vi "SPI Master and Slave with debug and disconnect [FPGA].vi"() -> ()   [LabVIEW 2011]
uses:
  <vilib>/Platform/TimedLoop/XDataNode/timing_clust.ctl
  <vilib>/Platform/TimedLoop/XDataNode/nitl_modes.ctl
  <vilib>/Platform/TimedLoop/XDataNode/wakeup.ctl
  SPI Slave State.ctl
  SPI Master State.ctl
  <vilib>/rvi/interface/RandomDataEmulation/nirviRandomDataFPGAFIFO.vi
  <vilib>/rvi/interface/RandomDataEmulation/niFpgaRandomDataHandleErrors.vi
  <vilib>/Platform/TimedLoop/XDataNode/XDataNode.xnode
  <vilib>/rvi/DataTransferAndStorage/Container/XNode/niFpgaContainer.xnode
  <vilib>/rvi/interface/RandomDataEmulation/nirviRandomDataFpgaReadWriteTemplate.vi
  <vilib>/Platform/TimedLoop/XDataNode/XDNodeRunTimeDep.lvlib
panel:
  in  "Disconnect Master and Slave":bool
  out "Slave Data Out":u32
  in  "Slave Data In":u32
  in  "Data Length":u8
  in  "HCP-1":u8
  out "Data Out":u32
  in  "Data In":u32
  in  "TX":bool
  in  "CPOL":bool
  in  "CPHA":bool
  in  "RESET":bool
  out "_SS":bool
  out "SCLK":bool
  out "MOSI":bool
  out "MISO":bool
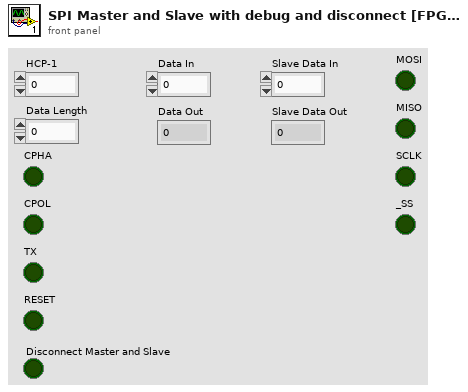
[diagram p1: front panel]
types:
  T1 = typedef "XDNodeRunTimeDep.lvlib/timing_clust.ctl" = cluster{"Expected End [f-1]":u64, "Actual End [f-1]":u64, "Finished Late? [f-1]":bool, "Expected End [i-1]":u64, "Actual End [i-1]":u64, "Finished Late? [i-1]":bool, "Expected Start [i]":u64, "Actual Start [i]":u64, "Expected Start [f]":u64, "Actual Start [f]":u64, "Source Name":string, "Structure Name":string, "Period":i64, "Deadline":i64, "Offset":i64, "Start":i64, "Priority":i32, "Timeout":i32, "Mode":T2, "Wakeup Reason":T3, "Error":errorcluster, "Source Type":string, "Secondary Source Type":string, "Global End Time":u64, "Global Start Time":u64, "Frame Duration":u64, "Iteration Duration":u64, "Assigned CPU":i32, "I/O Scan Engine Mode":u32}
  T2 = typedef "XDNodeRunTimeDep.lvlib/nitl_modes.ctl" = enum32{"No Change", "Process missed periods, maintain original phase", "Discard missed periods, maintain original phase", "Process missed periods, ignore original phase", "Discard missed periods, ignore original phase"}
  T3 = typedef "XDNodeRunTimeDep.lvlib/wakeup.ctl" = enum32{"Normal", "Aborted", "Asynchronous wakeup", "Timing source error", "Timed loop error", "Timeout"}
  T4 = typedef "SPI Slave State.ctl" = enum8{"RESET", "Wait for _SS", "Assert MISO", "Latch MOSI"}
  T5 = typedef "SPI Master State.ctl" = enum8{"RESET", "Wait for TX", "Assert MOSI", "Toggle SCLK", "Latch MISO and Toggle SCLK", "Assert MOSI and Toggle SCLK"}
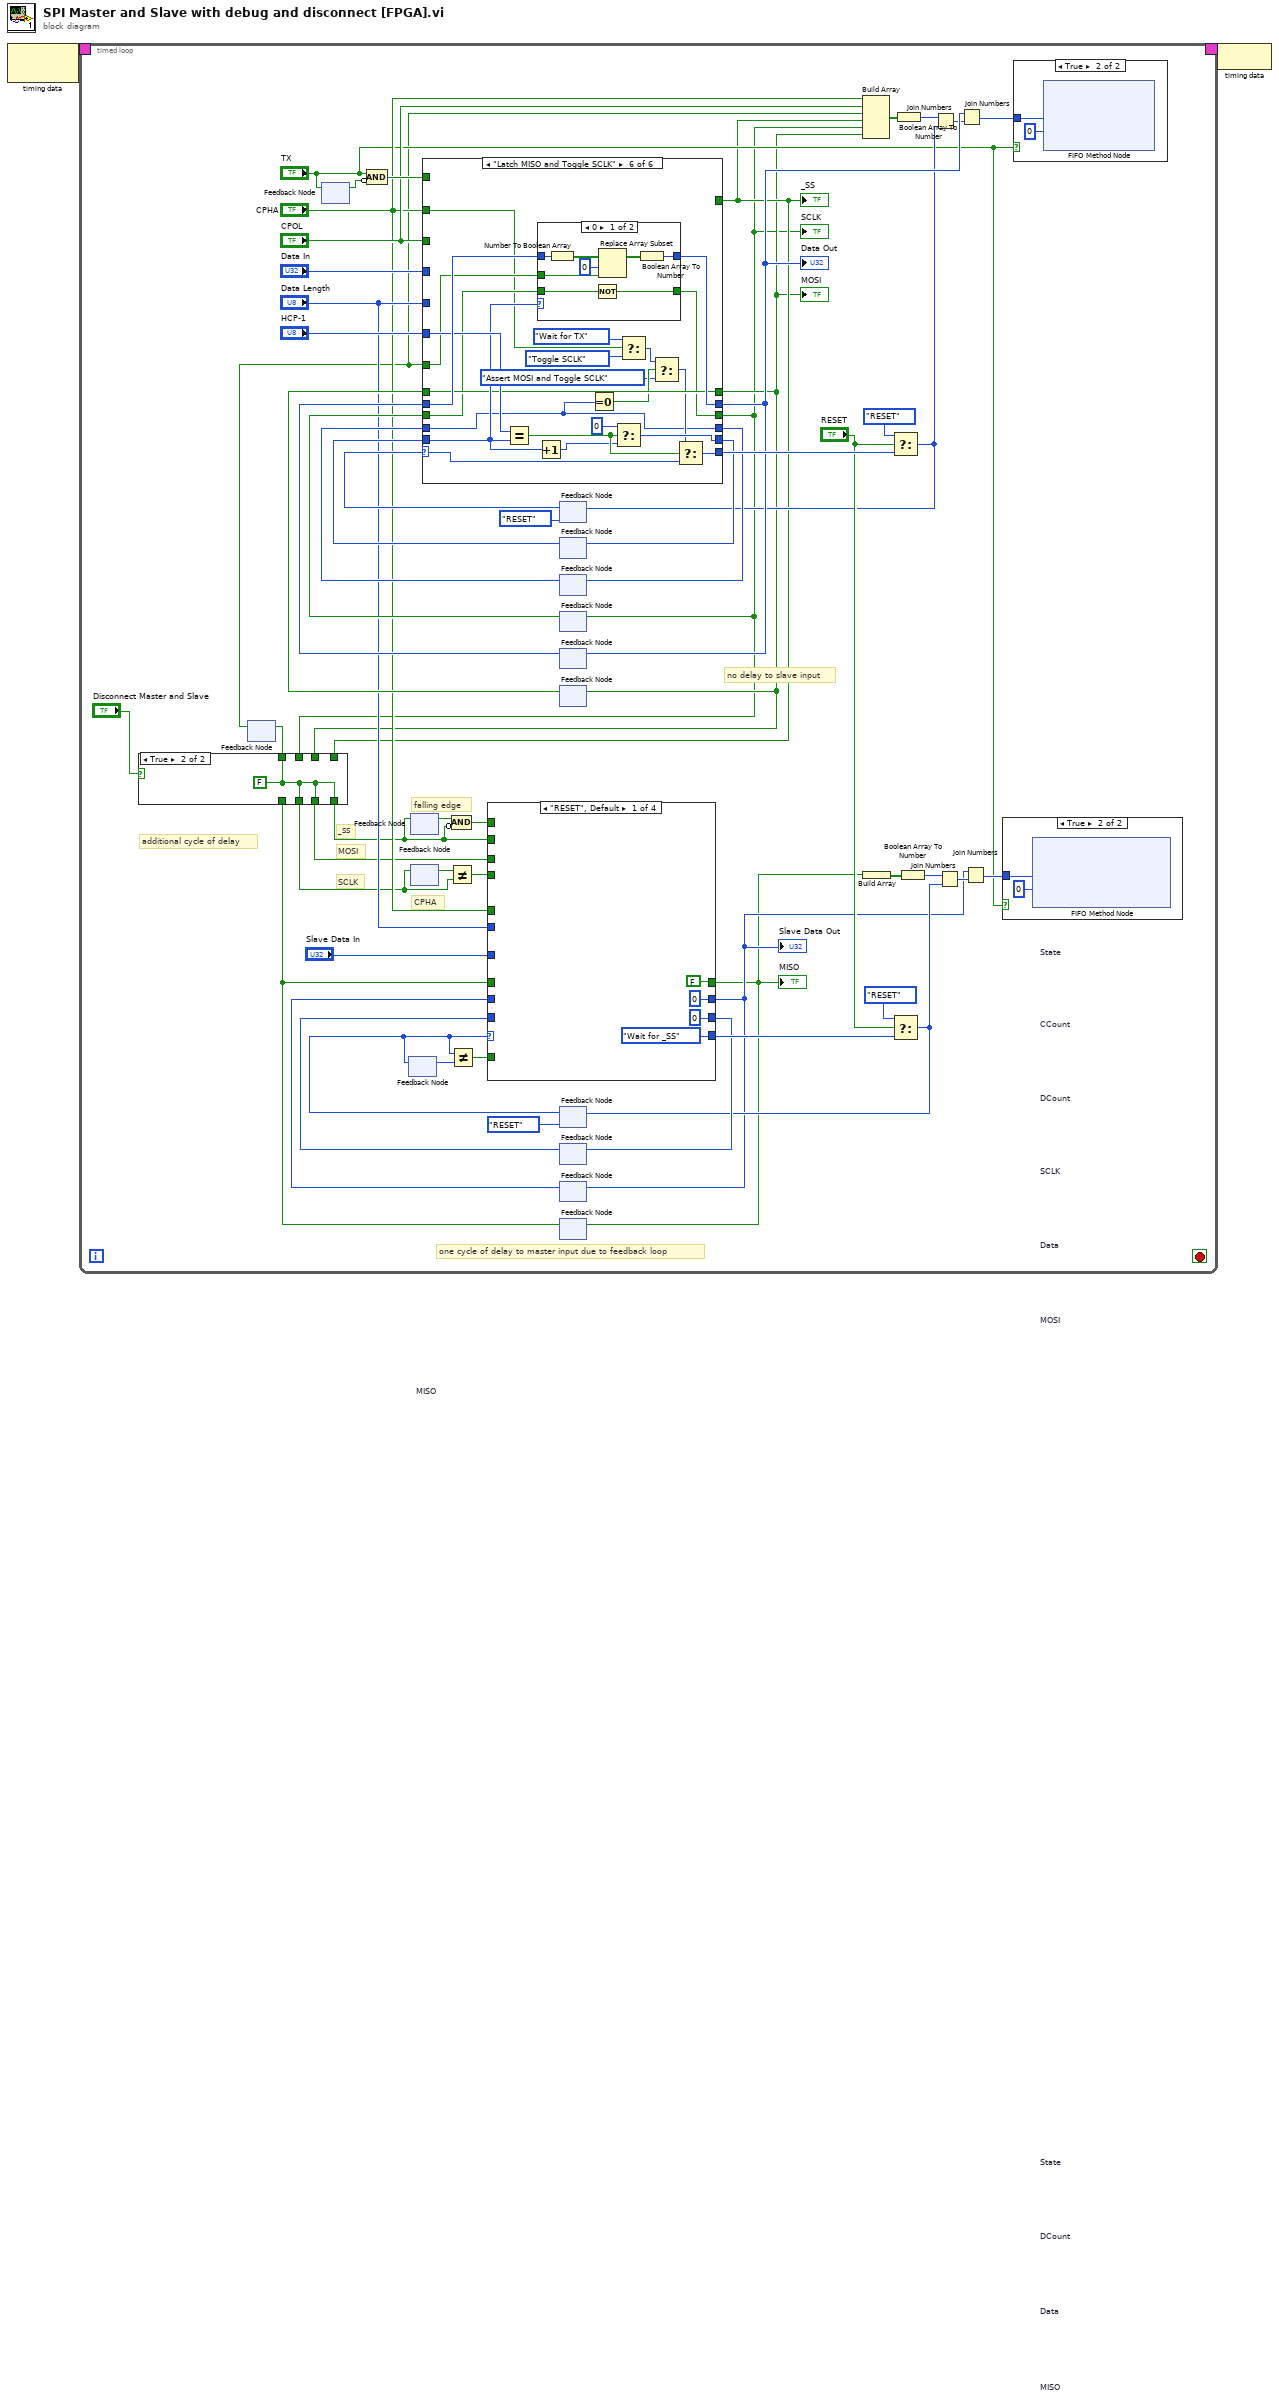
[diagram p0: block diagram]
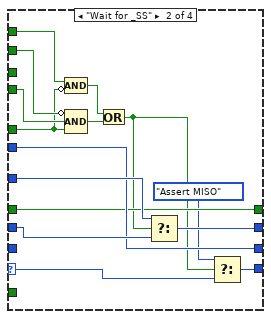
[diagram p4: hidden frame]
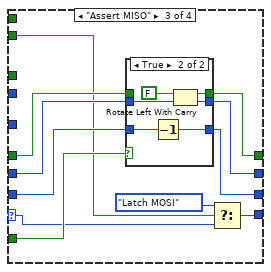
[diagram p5: hidden frame]
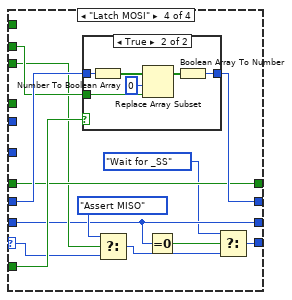
[diagram p7: hidden frame]
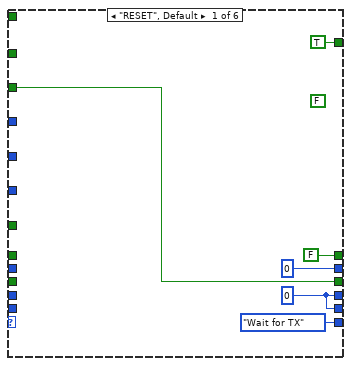
[diagram p10: hidden frame]
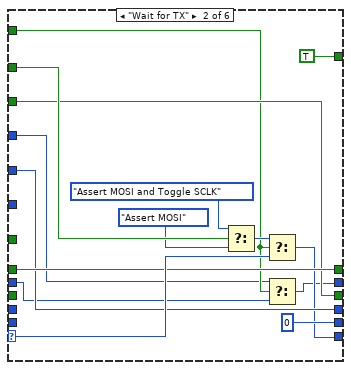
[diagram p11: hidden frame]
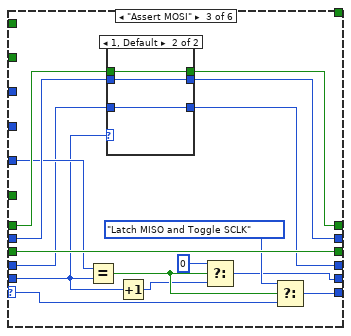
[diagram p12: hidden frame]
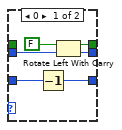
[diagram p13: hidden frame]
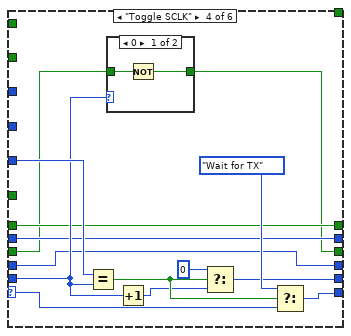
[diagram p14: hidden frame]
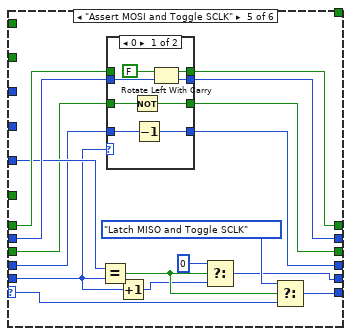
[diagram p16: hidden frame]
diagram:
  n1 = node-c288() -> (w2:T1)  [unwired: 1 in]
  n2 = timed-loop {
    timing: w2 -> [_]
    timing-out: [_] -> w1
    stop <- _ stop-if-true
    # "additional cycle of delay"
    # "CPHA"
    # "falling edge"
    # "SCLK"
    # "MOSI"
    # "_SS"
    # "one cycle of delay to master input due to feedback loop"
    # "no delay to slave input"
    n3 = feedback #1 "MISO"() -> (w7:bool)  [unwired: 1 in]
    n4 = feedback #2() -> (w55:bool)  [unwired: 1 in]
    n5 = feedback-in #2("TX") -> ()
    n6 = Compound Arithmetic op=AND("TX", invert w55) -> (w47:bool)
    n7 = feedback #3 ("State")() -> (w23:T4)  [unwired: 1 in]
    n8 = feedback #4() -> (w27:bool)  [unwired: 1 in]
    n9 = feedback #5() -> (w25:bool)  [unwired: 1 in]
    n10 = feedback #6 "State"(SPI_Master_State."RESET") -> (w58:T5)
    n11 = feedback #7 "CCount"() -> (w52:u8)  [unwired: 1 in]
    n12 = feedback #8 "DCount"() -> (w51:u8)  [unwired: 1 in]
    n13 = feedback #9 "SCLK"() -> (w50:bool)  [unwired: 1 in]
    n14 = feedback #10 "Data"() -> (w48:u32)  [unwired: 1 in]
    n15 = feedback #11 "MOSI"() -> (w46:bool)  [unwired: 1 in]
    n16 = case shown="\"Latch MISO and Toggle SCLK\"" w58 {
      selector: w58 -> [_ w145 w157 w185 w201 w237]
      tunnel: [SPI_Master_State."Wait for TX" w138 w158 w186 w202 w238] -> w57
      tunnel: w47 -> [_ w137 _ _ _ _]
      tunnel: [w132 u8 0 w151 w179 w195 w232] -> w54
      tunnel: [w132 w140 w149 w178 w191 w220] -> w53
      tunnel: w52 -> [_ _ w154 w182 w198 w235]
      tunnel: w51 -> [_ _ w150 w178 w192 w220]
      tunnel: [TRUE ("MOSI") TRUE ("MOSI") _ _ _ _] -> w12
      tunnel: "CPHA" -> [_ w146 _ _ _ w226]
      tunnel: [w130 w139 w160 w174 w193 w228] -> w10
      tunnel: "CPOL" -> [w130 w139 _ _ _ _]
      tunnel: w50 -> [_ _ w160 w175 w194 w229]
      tunnel: "Data In" -> [_ w136 _ _ _ _]
      tunnel: [u32 0 ("Data In") w134 w163 w177 w206 w240] -> w40
      tunnel: w48 -> [_ w135 w164 w177 w207 w241]
      tunnel: "HCP-1" -> [_ _ w159 w187 w203 w239]
      tunnel: w7 -> [_ _ _ _ _ w230]
      tunnel: "Data Length" -> [_ w140 _ _ _ _]
      tunnel: [FALSE ("msb carry out") w141 w162 w176 w205 w231] -> w11
      tunnel: w46 -> [_ w141 w161 w176 w204 w231]
      frame "RESET", Default {
        (unwired) FALSE ("msb carry out")
        w132 = u8 0
      }
      frame "Wait for TX" {
        n17 = Select(t=SPI_Master_State."Assert MOSI and Toggle SCLK", s=w146, f=SPI_Master_State."Assert MOSI" ("t")) -> (s? t:f=w142:T5)
        n18 = Select(t=w142, s=w137, f=w145) -> (s? t:f=w138:T5)
        n19 = Select(t=w136, s=w137, f=w135) -> (s? t:f=w134:u32)
      }
      frame "Assert MOSI" {
        n20 = Equal?(x=w159, y=w154) -> (x = y?=w155:bool)
        n21 = case shown="1, Default" w154 {
          tunnel: w164 -> [w169 w172]
          tunnel: [w168 w172] -> w163
          tunnel: [w167 w173] -> w162
          tunnel: w161 -> [_ w173]
          tunnel: w150 -> [w166 w171]
          tunnel: [w165 w171] -> w149
          frame 0 {
            n22 = Decrement(x=w166) -> (x-1=w165:u8)
            n23 = Rotate Left With Carry(2:w169, 3:FALSE ("carry")) -> (0:w168:u32, 1:w167:bool)
          }
          frame 1, Default {
          }
        }
        n24 = Increment(x=w154) -> (x+1=w153:u8)
        n25 = Select(t=u8 0, s=w155, f=w153) -> (s? t:f=w151:u8)
        n26 = Select(t=SPI_Master_State."Latch MISO and Toggle SCLK", s=w155, f=w157) -> (s? t:f=w158:T5)
      }
      frame "Toggle SCLK" {
        n27 = Equal?(x=w187, y=w182) -> (x = y?=w183:bool)
        n28 = case shown="0" w182 {
          tunnel: w175 -> [w189 w190]
          tunnel: [w188 w190] -> w174
          frame 0 {
            n29 = Not(x=w189) -> (.not. x?=w188:bool)
          }
          frame 1, Default {
          }
        }
        n30 = Increment(x=w182) -> (x+1=w181:u8)
        n31 = Select(t=u8 0, s=w183, f=w181) -> (s? t:f=w179:u8)
        n32 = Select(t=SPI_Master_State."Wait for TX", s=w183, f=w185) -> (s? t:f=w186:T5)
      }
      frame "Assert MOSI and Toggle SCLK" {
        n33 = Equal?(x=w203, y=w198) -> (x = y?=w199:bool)
        n34 = case shown="0" w198 {
          tunnel: w207 -> [w214 w218]
          tunnel: [w213 w218] -> w206
          tunnel: [w212 w219] -> w205
          tunnel: w204 -> [_ w219]
          tunnel: w194 -> [w211 w217]
          tunnel: [w210 w217] -> w193
          tunnel: w192 -> [w209 w216]
          tunnel: [w208 w216] -> w191
          frame 0 {
            n35 = Not(x=w211) -> (.not. x?=w210:bool)
            n36 = Decrement(x=w209) -> (x-1=w208:u8)
            n37 = Rotate Left With Carry(2:w214, 3:FALSE ("carry")) -> (0:w213:u32, 1:w212:bool)
          }
          frame 1, Default {
          }
        }
        n38 = Increment(x=w198) -> (x+1=w197:u8)
        n39 = Select(t=u8 0, s=w199, f=w197) -> (s? t:f=w195:u8)
        n40 = Select(t=SPI_Master_State."Latch MISO and Toggle SCLK", s=w199, f=w201) -> (s? t:f=w202:T5)
      }
      frame "Latch MISO and Toggle SCLK" {
        n41 = Equal?(x=w239, y=w235) -> (x = y?=w236:bool)
        n42 = Increment(x=w235) -> (x+1=w234:u8)
        n43 = case shown="0" w235 {
          tunnel: w241 -> [w249 w251]
          tunnel: [w244 w251] -> w240
          tunnel: w230 -> [w247 _]
          tunnel: w229 -> [w243 w250]
          tunnel: [w242 w250] -> w228
          frame 0 {
            n44 = Number To Boolean Array(number=w249) -> (Boolean array=w248:bool[])
            n45 = Not(x=w243) -> (.not. x?=w242:bool)
            n46 = Replace Array Subset(array=w248, new element=w247, index=0) -> (w245:bool[])
            n47 = Boolean Array To Number(Boolean array=w245) -> (number=w244:u32)
          }
          frame 1, Default {
          }
        }
        n48 = Equal To 0?(x=w220) -> (x = 0?=w227:bool)
        n49 = Select(t=u8 0, s=w236, f=w234) -> (s? t:f=w232:u8)
        n50 = Select(t=SPI_Master_State."Wait for TX", s=w226, f=SPI_Master_State."Toggle SCLK" ("t")) -> (s? t:f=w222:T5)
        n51 = Select(t=w222, s=w227, f=SPI_Master_State."Assert MOSI and Toggle SCLK" ("t")) -> (s? t:f=w224:T5)
        n52 = Select(t=w224, s=w236, f=w237) -> (s? t:f=w238:T5)
      }
    }
    "SCLK" <- w10
    "_SS" <- w12
    "MOSI" <- w11
    "Data Out" <- w40
    n53 = feedback-in #7(w54) -> ()
    n54 = feedback-in #8(w53) -> ()
    n55 = feedback-in #9(w10) -> ()
    n56 = feedback-in #10(w40) -> ()
    n57 = feedback-in #11(w11) -> ()
    n58 = feedback #12 "State"(SPI_Slave_State."RESET" ("SPI Slave State")) -> (w22:T4)
    n59 = feedback-in #3(w22) -> ()
    n60 = Not Equal?(x=w22, y=w23) -> (x != y?=w21:bool)
    n61 = feedback #13 "DCount"() -> (w34:u8)  [unwired: 1 in]
    n62 = feedback #14 "Data"() -> (w31:u32)  [unwired: 1 in]
    n63 = feedback #15 "MISO"() -> (w9:bool)  [unwired: 1 in]
    n64 = case shown="True" "Disconnect Master and Slave" {
      tunnel: w12 -> [w63 _]
      tunnel: [w63 w64] -> w4
      tunnel: w11 -> [w62 _]
      tunnel: [w62 w64] -> w5
      tunnel: w10 -> [w61 _]
      tunnel: [w61 w64] -> w6
      tunnel: w9 -> [w60 _]
      tunnel: [w60 w64] -> w8
      frame False {
      }
      frame True {
        w64 = FALSE ("msb carry out")
      }
    }
    n65 = feedback-in #1(w8) -> ()
    n66 = feedback-in #4(w4) -> ()
    n67 = feedback-in #5(w6) -> ()
    n68 = Not Equal?(x=w25, y=w6) -> (x != y?=w24:bool)
    n69 = Compound Arithmetic op=AND(w27, invert w4) -> (w26:bool)
    n70 = case shown="\"RESET\", Default" w22 {
      selector: w22 -> [_ w73 w89 w112]
      tunnel: w5 -> [_ _ _ w115]
      tunnel: [SPI_Slave_State."Wait for _SS" ("SPI Slave State") w78 w88 w109] -> w37
      tunnel: w4 -> [_ w85 _ _]
      tunnel: w34 -> [_ _ w93 w108]
      tunnel: [u8 0 w79 w92 w108] -> w33
      tunnel: [u32 0 ("Data In") w81 w91 w116] -> w14
      tunnel: w31 -> [_ w80 w95 w118]
      tunnel: w9 -> [_ w76 w94 w114]
      tunnel: [FALSE ("msb carry out") w76 w90 w114] -> w13
      tunnel: "Data Length" -> [_ w79 _ _]
      tunnel: "Slave Data In" -> [_ w82 _ _]
      tunnel: "CPHA" -> [_ w71 _ _]
      tunnel: w26 -> [_ w83 _ _]
      tunnel: w24 -> [_ w84 w87 w113]
      tunnel: w21 -> [_ _ w96 w117]
      frame "RESET", Default {
      }
      frame "Wait for _SS" {
        n71 = Compound Arithmetic op=AND(w83, invert w71) -> (w74:bool)
        n72 = Compound Arithmetic op=AND(invert w85, w84, w71) -> (w77:bool)
        n73 = Or(x=w74, y=w77) -> (x .or. y?=w72:bool)
        n74 = Select(t=w82, s=w72, f=w80) -> (s? t:f=w81:u32)
        n75 = Select(t=SPI_Slave_State."Assert MISO", s=w72, f=w73) -> (s? t:f=w78:T4)
      }
      frame "Assert MISO" {
        n76 = case shown="True" w96 {
          tunnel: w95 -> [w98 w104]
          tunnel: [w98 w103] -> w91
          tunnel: [w99 w102] -> w90
          tunnel: w94 -> [w99 _]
          tunnel: w93 -> [w97 w101]
          tunnel: [w97 w100] -> w92
          frame False {
          }
          frame True {
            n77 = Decrement(x=w101) -> (x-1=w100:u8)
            n78 = Rotate Left With Carry(2:w104, 3:FALSE ("carry")) -> (0:w103:u32, 1:w102:bool)
          }
        }
        n79 = Select(t=SPI_Slave_State."Latch MOSI", s=w87, f=w89) -> (s? t:f=w88:T4)
      }
      frame "Latch MOSI" {
        n80 = case shown="True" w117 {
          tunnel: w118 -> [w119 w125]
          tunnel: [w119 w120] -> w116
          tunnel: w115 -> [_ w123]
          frame False {
          }
          frame True {
            n81 = Number To Boolean Array(number=w125) -> (Boolean array=w124:bool[])
            n82 = Replace Array Subset(array=w124, new element=w123, index=0) -> (w121:bool[])
            n83 = Boolean Array To Number(Boolean array=w121) -> (number=w120:u32)
          }
        }
        n84 = Select(t=SPI_Slave_State."Assert MISO", s=w113, f=w112) -> (s? t:f=w110:T4)
        n85 = Equal To 0?(x=w108) -> (x = 0?=w107:bool)
        n86 = Select(t=SPI_Slave_State."Wait for _SS", s=w107, f=w110) -> (s? t:f=w109:T4)
      }
    }
    "MISO" <- w13
    "Slave Data Out" <- w14
    n87 = feedback-in #13(w33) -> ()
    n88 = feedback-in #14(w14) -> ()
    n89 = feedback-in #15(w13) -> ()
    n90 = Build Array("CPHA", "CPOL", w7, w12, w10, w11) -> (w42:bool[])
    n91 = Build Array(w13) -> (w18:bool[])
    n92 = Select(t=SPI_Master_State."RESET", s="RESET", f=w57) -> (s? t:f=w32:T5)
    n93 = feedback-in #6(w32) -> ()
    n94 = Select(t=SPI_Slave_State."RESET", s="RESET", f=w37) -> (s? t:f=w16:T4)
    n95 = feedback-in #12(w16) -> ()
    n96 = Boolean Array To Number(Boolean array=w42) -> (number=w41:u8)
    n97 = Boolean Array To Number(Boolean array=w18) -> (number=w19:u8)
    n98 = Join Numbers(hi=w41, lo=w32) -> ((hi.lo)=w39:u16)
    n99 = Join Numbers(hi=w19, lo=w16) -> ((hi.lo)=w20:u16)
    n100 = Join Numbers(hi=w40, lo=w39) -> ((hi.lo)=w44:u64)
    n101 = Join Numbers(hi=w14, lo=w20) -> ((hi.lo)=w17:u64)
    n102 = case shown="True" "TX" {
      tunnel: w17 -> [_ w65]
      frame False {
      }
      frame True {
        n103 = xnode ("FIFO Method Node")("Element"=w65, "Timeout"=0) -> ()  [unwired: 1 in, 2 out]
      }
    }
    n104 = case shown="True" "TX" {
      tunnel: w44 -> [_ w126]
      frame False {
      }
      frame True {
        n105 = xnode ("FIFO Method Node")("Element"=w126, "Timeout"=0) -> ()  [unwired: 1 in, 2 out]
      }
    }
  }
  n106 = node-c288(w1) -> ()
